vi "lvEtherbone.application_example_read.vi"() -> ()   [LabVIEW 2009, in "lvEtherbone.lvlib"]
doc: "This example performs a simple read cycle on a Etherbone device."
uses:
  lvEtherbone.lvlib
panel:
  out "data":u64 format="%.0x"
  in  "timeout [ms]":i32=1000
  in  "address":u64=32768 format="%.0x"
  in  "ip_port":string="111.222.333.444:5555"
  out "error out":errorcluster
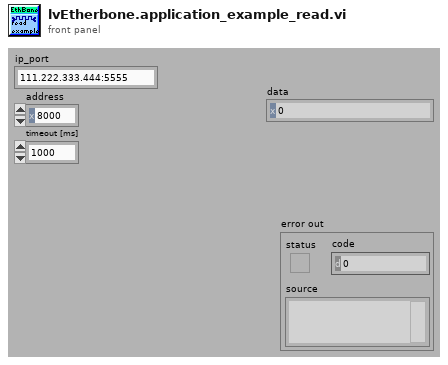
[diagram p1: front panel]
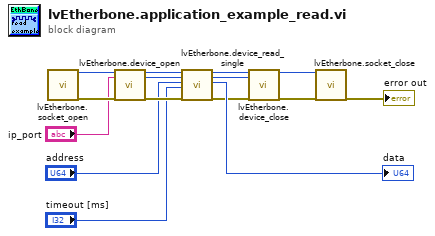
[diagram p0: block diagram]
diagram:
  n1 = call "lvEtherbone.socket_open.vi"() -> ("eb_socket_ID"=w13:i32, "error out"=w14:errorcluster)  [unwired: 17 in, 1 out]
  n2 = call "lvEtherbone.device_open.vi"("eb_socket_ID"=w13, "ip_port"="ip_port", "error in (no error)"=w14) -> ("eb_socket_ID out"=w5:i32, "eb_device_ID"=w11:i32, "error out"=w12:errorcluster)  [unwired: 13 in, 1 out]
  n3 = call "lvEtherbone.device_read_single.vi"("eb_socket_ID"=w5, "eb_device_ID"=w11, "address"="address", "timeout [ms]"="timeout [ms]", "error in (no error)"=w12) -> ("eb_socket_ID out"=w1:i32, "eb_device_ID out"=w3:i32, "data"=→"data":u64, "error out"=w2:errorcluster)  [unwired: 9 in, 2 out]
  n4 = call "lvEtherbone.device_close.vi"("eb_socket_ID"=w1, "eb_device_ID"=w3, "error in (no error)"=w2) -> ("eb_socket_ID out"=w4:i32, "error out"=w10:errorcluster)  [unwired: 14 in, 1 out]
  n5 = call "lvEtherbone.socket_close.vi"("eb_socket_ID"=w4, "error in (no error)"=w10) -> ("error out"=→"error out":errorcluster)  [unwired: 16 in, 1 out]
